vi "Hydra TVS Test.vi"(8 "error out":errorcluster) -> (0 "error out 2":errorcluster, 3 "Boolean":bool)   [LabVIEW 2022 SP3]
panel:
  out "Result (color)":u32(colorbox)
  out "Instructional Message":string
  in  "OK Button":bool
  in  "bypass":bool
  in  "stop":bool
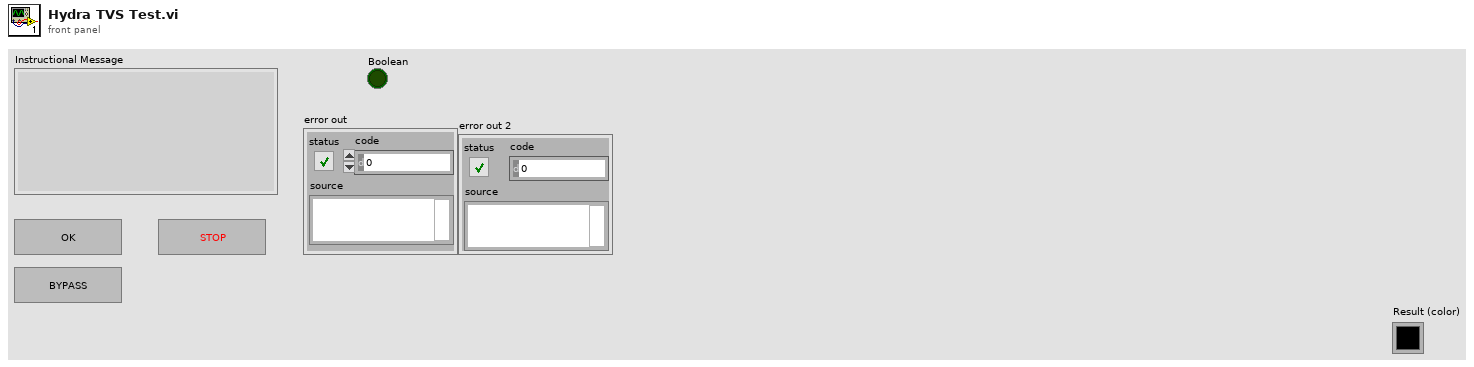
[diagram p1: front panel]
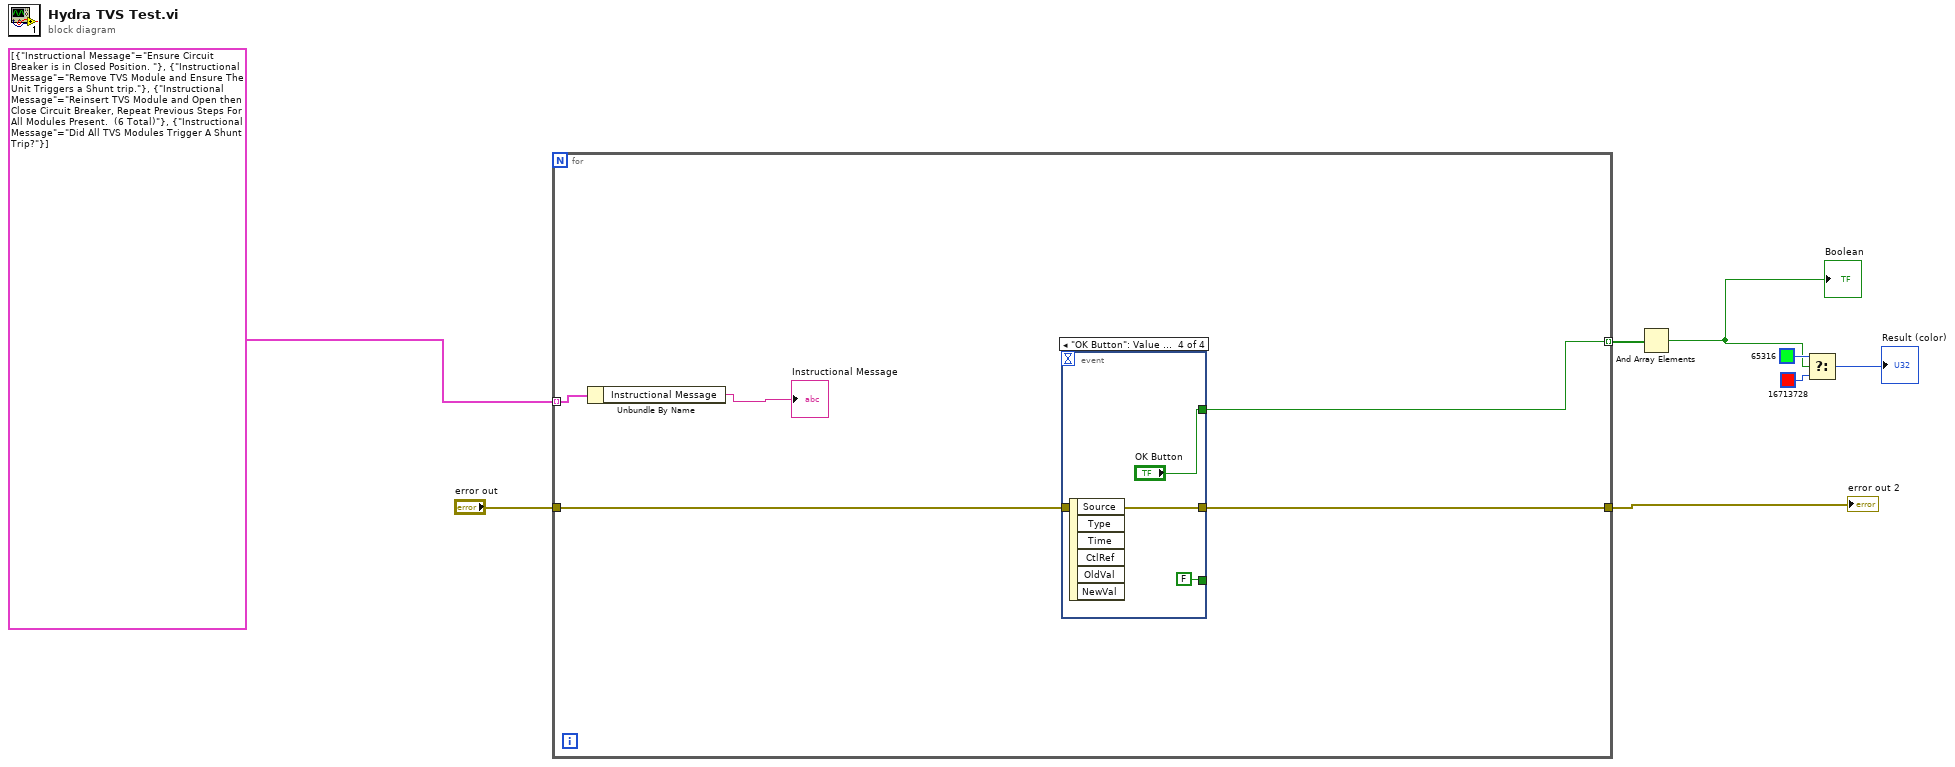
[diagram p0: block diagram]
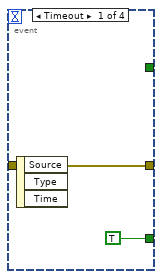
[diagram p2: hidden frame]
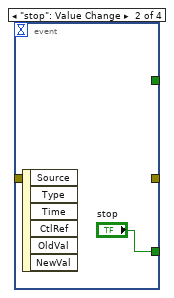
[diagram p3: hidden frame]
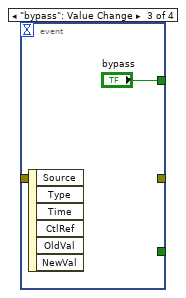
[diagram p4: hidden frame]
diagram:
  n1 = for {
    tunnel: cluster{"Instructional Message":string}[] [{"Instructional Message"="Ensure Circuit Breaker is in Closed Position. "}, {"Instructional Message"="Remove TVS Module and Ensure The Unit Triggers a Shunt trip."}, {"Instructional Message"="Reinsert TVS Module and Open then Close Circuit Breaker, Repeat Previous Steps For All Modules Present.  (6 Total)"}, {"Instructional Message"="Did All TVS Modules Trigger A Shunt Trip?"}] -> [w10] mode=indexing
    tunnel: "error out" -> [w13]
    tunnel: [w11] -> w3
    tunnel: [w9] -> w2 mode=indexing
    n2 = Unbundle By Name(w10) -> ("Instructional Message"=→"Instructional Message":string)
    n3 = event shown="[3] \"OK Button\": Value Change" {
      selector: _ -> [_ _ _ _]
      dyn-events: _ -> [_ _ _ _]
      timeout: _ -> [_ _ _ _]
      tunnel: w13 -> [w15 _ _ w20]
      tunnel: [w15 _ _ w20] -> w11
      tunnel: [TRUE "stop" _ FALSE] -> _
      tunnel: [_ _ "bypass" "OK Button"] -> w9
      event Timeout {
        n4 = event-data() -> ()  [unwired: 1 in, 3 out]
      }
      event "stop": Value Change {
        n5 = event-data() -> ()  [unwired: 1 in, 6 out]
      }
      event "bypass": Value Change {
        n6 = event-data() -> ()  [unwired: 1 in, 6 out]
      }
      event "OK Button": Value Change {
        n7 = event-data() -> ()  [unwired: 1 in, 6 out]
      }
    }
  }
  "error out 2" <- w3
  n8 = And Array Elements(Boolean array=w2) -> (logical AND=w1:bool)
  "Boolean" <- w1
  n9 = Select(t=u32 65316 ("Result (color)"), s=w1, f=u32 16713728 ("Result (color)")) -> (s? t:f=→"Result (color)":u32)
